vi "DAQ_AngleToVolt.vi"(11 "Angle":dbl) -> (3 "Voltage":dbl)   [LabVIEW 2022 SP3]
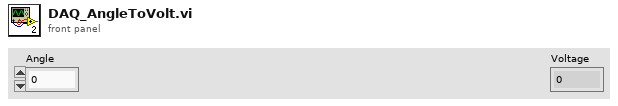
[diagram p1: front panel]
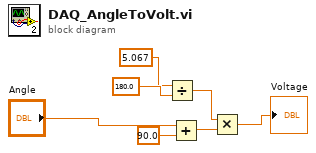
[diagram p0: block diagram]
diagram:
  n1 = Divide(x=5.067 ("y"), y=180.0 ("x")) -> (x/y=w2:dbl)
  n2 = Add(x="Angle", y=90.0) -> (x+y=w3:dbl)
  n3 = Multiply(x=w2, y=w3) -> (x*y=→"Voltage":dbl)
